vi "Sine wave and Frequency exercise.vi"() -> ()   [LabVIEW 2024]
uses:
  <vilib>/measure/NI_MABase.lvlib
panel:
  in  "sampling info 2":cluster{"Fs":dbl, "#s":dbl}={"Fs"=1000.0, "#s"=1000.0} {"Fs" format="%.2p"}
  in  "amplitude 2":dbl=1.0 format="%0.2p"
  in  "phase 2":dbl format="%.2p"
  in  "frequency 2":dbl=10.0 format="%0.2p"
  in  "sampling info":cluster{"Fs":dbl, "#s":dbl}={"Fs"=1000.0, "#s"=1000.0} {"Fs" format="%.2p"}
  out "Waveform Graph":waveform(dbl)[](graph)
  in  "amplitude":dbl=1.0 format="%0.2p"
  in  "phase":dbl format="%.2p"
  in  "frequency":dbl=10.0 format="%0.2p"
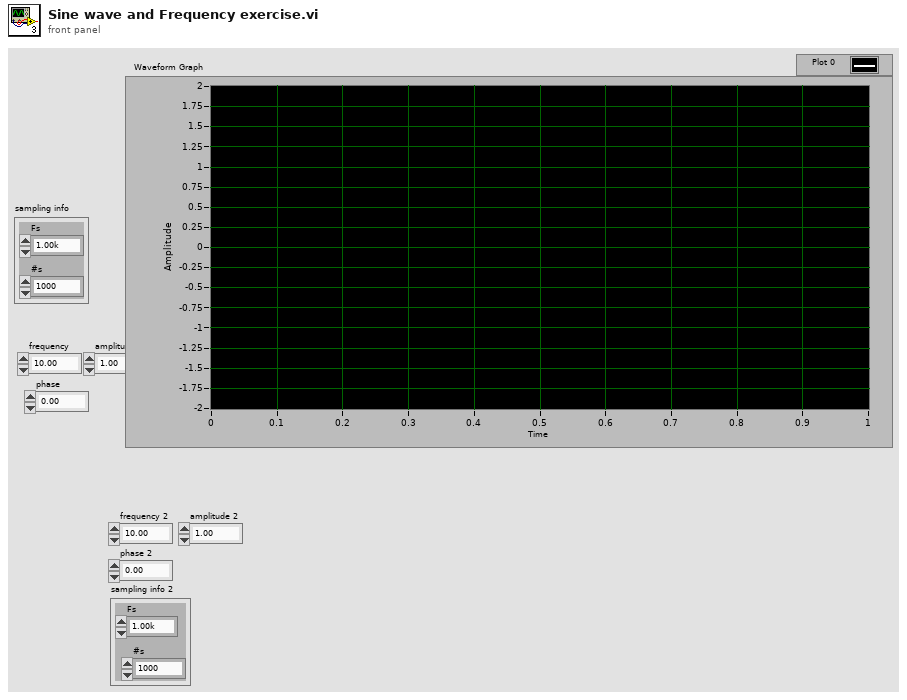
[diagram p1: front panel]
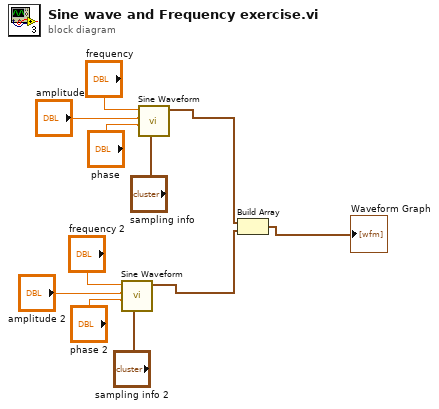
[diagram p0: block diagram]
diagram:
  n1 = call <vilib>:"Sine Waveform.vi"("sampling info"="sampling info 2", "phase"="phase 2", "amplitude"="amplitude 2", "frequency"="frequency 2") -> ("signal out"=w3:waveform(dbl))  [unwired: 6 in, 1 out]
  n2 = call <vilib>:"Sine Waveform.vi"("sampling info"="sampling info", "phase"="phase", "amplitude"="amplitude", "frequency"="frequency") -> ("signal out"=w2:waveform(dbl))  [unwired: 6 in, 1 out]
  n3 = Build Array(w2, w3) -> (→"Waveform Graph":waveform(dbl)[])
